vi "Read (Multiple Points).vi"(7 "Maximum Time (10000 ms)":u32=10000, 8 "error in (no error)":errorcluster, 9 "Number of Points (100)":u32=100, 10 "Channel (1: Channel 1 Display)":u16(ring)=1 items=["Channel 1 Display"=1, "Channel 2 Display"=2], 11 "VISA resource name":refnum<visa-resource-name>) -> (0 "error out":errorcluster, 2 "Measurements":sgl[](array[numeric]), 3 "VISA resource name out":refnum<visa-resource-name>)   [LabVIEW 2012, in "Stanford Research 830.lvlib"]
doc: "Reads the values of the selected channel display on the instrument.\n\n<B>Note:</B>\n\nThis VI retrieves the actual value of the Channel Display, not the value of the physical channel output.\n\nChannel Display is configured in <B>Configure Channel Display.vi</B>"
uses:
  Stanford Research 830.lvlib
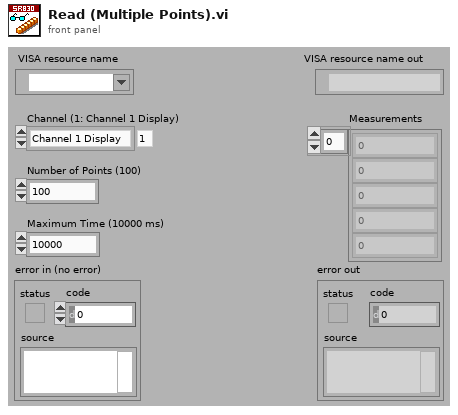
[diagram p1: front panel]
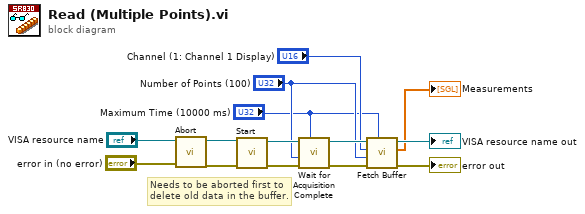
[diagram p0: block diagram]
diagram:
  # "Needs to be aborted first to delete old data in the buffer."
  n1 = call "Abort.vi"("error in (no error)"="error in (no error)", "VISA resource name"="VISA resource name") -> ("error out"=w3:errorcluster, "VISA resource name out"=w4:refnum<visa-resource-name>)  [unwired: 8 in]
  n2 = call "Start.vi"("error in (no error)"=w3, "VISA resource name"=w4) -> ("error out"=w13:errorcluster, "VISA resource name out"=w14:refnum<visa-resource-name>)  [unwired: 8 in]
  n3 = call "Wait for Acquisition Complete.vi"("Maximum Time (10000 ms)"="Maximum Time (10000 ms)", "error in (no error)"=w13, "Number of Points (100)"="Number of Points (100)", "VISA resource name"=w14) -> ("error out"=w11:errorcluster, "VISA resource name out"=w12:refnum<visa-resource-name>)  [unwired: 6 in]
  n4 = call "Fetch Buffer.vi"("Timeout (10000 ms)"="Maximum Time (10000 ms)", "error in (no error)"=w11, "Number of Points (100)"="Number of Points (100)", "Channel (1: Channel 1 Display)"="Channel (1: Channel 1 Display)", "VISA resource name"=w12) -> ("error out"=→"error out":errorcluster, "Measurements"=→"Measurements":sgl[], "VISA resource name out"=→"VISA resource name out":refnum<visa-resource-name>)  [unwired: 4 in]
